vi "Lvi Subsystem Set Ctr Cont Measure Mode.vi"(8 "error in (no error)":errorcluster, 9 "StopEdge":i32, 10 "StartEdge":i32, 11 "TaskRef":i32) -> (0 "error out":errorcluster, 2 "function return":i32, 3 "TaskRef out":i32)   [LabVIEW 2016, in "DtLvLink.lvlib"]
doc: "Calls directly into the entry points of the DLL of the Data Acq SDK to create one or more virtual channels, add them to a task, and configure the task with the specified settings to measure the time, in milliseconds, between a specified start edge and stop edge of the counter's clock or gate input signal. This VI automatically restarts the next measurement. This VI is used by the higher-level VI, DtOLCreateTask."
uses:
  <userlib>/LV-Link3/DtLvLink.lvlib
  <userlib>/LV-Link3/DtLvLink_32.dll
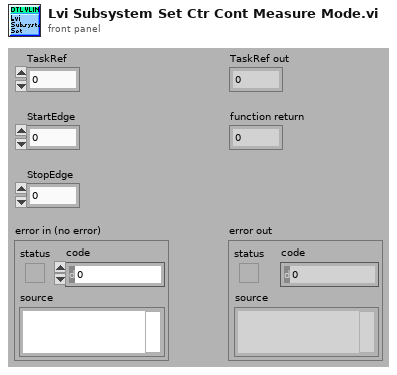
[diagram p1: front panel]
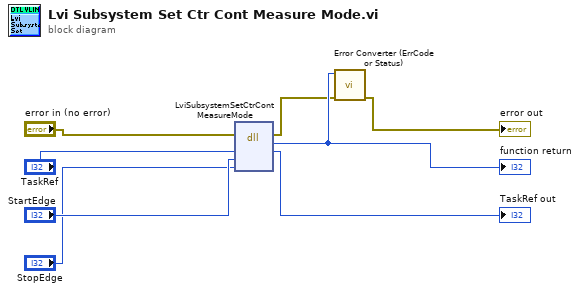
[diagram p0: block diagram]
diagram:
  n1 = dll-call lib="C:/Program Files (x86)/National Instruments/LabVIEW 2016/user.lib/LV-Link3/DtLvLink_32.*" fn="LviSubsystemSetCtrContMeasureMode"(error in="error in (no error)", "TaskRef"="TaskRef", "StartEdge"="StartEdge", "StopEdge"="StopEdge") -> (error out=w2:errorcluster, w8:i32, "TaskRef"=→"TaskRef out":i32)  [unwired: 4 in, 1 out]
  "function return" <- w8
  n2 = call <userlib>:"Error Converter (ErrCode or Status).vi"("error in (no error)"=w2, "error code"=w8) -> ("error out"=→"error out":errorcluster)  [unwired: 9 in]
